vi "Nominal Value Write Single.vi"(8 "error in":errorcluster, 9 "Channel Index":i32=1, 10 "Current Nominal Value":dbl, 11 "Current Nominal Value in":refnum<class "Current Nominal Value.lvclass">) -> (0 "error out":errorcluster, 3 "Current Nominal Value out":refnum<class "Current Nominal Value.lvclass">)   [LabVIEW 2023, in "Current Nominal Value.lvclass"]
uses:
  Current Nominal Value.lvclass
  Current Nominal Value.lvclass/Current Nominal Value.ctl
  Parents/Nominal Value/Nominal Value.lvclass
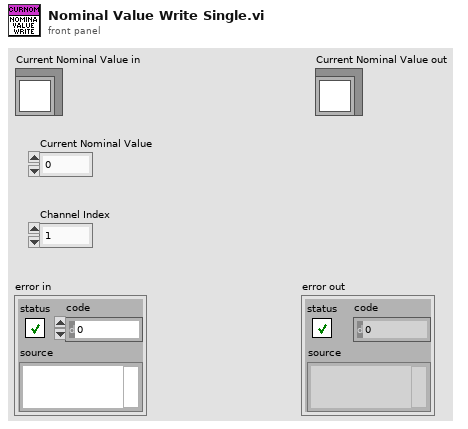
[diagram p1: front panel]
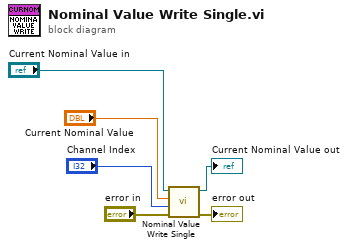
[diagram p0: block diagram]
diagram:
  n1 = call-parent "Nominal Value Write Single.vi"("error in"="error in", "Channel Index"="Channel Index", "Nominal Value"="Current Nominal Value", "Nominal Value in"="Current Nominal Value in") -> ("error out"=→"error out":errorcluster, "Nominal Value out"=→"Current Nominal Value out":refnum<class "Current Nominal Value.lvclass">)  [unwired: 6 in]
